vi "ajoutchambre.vi"() -> ()   [LabVIEW 2015]
uses:
  <vilib>/httpClient/LabVIEWHTTPClient.lvlib
panel:
  out "Tab Control 3":enum32{"Page 1", "Page 2"}(tab)
  out "Tab Control 2":enum32{"Page 1", "Page 2"}(tab)
  in  "desc":string
  in  "OK Button 4":bool
  in  "OK Button 2":bool
  out "Tab Control":enum32{"Page 1", "Page 2"}(tab)
  in  "nom":string
  in  "matricule":string
  # "Entrer Matricule"
  # "Entrer Nom"
  # "Entrer Description"
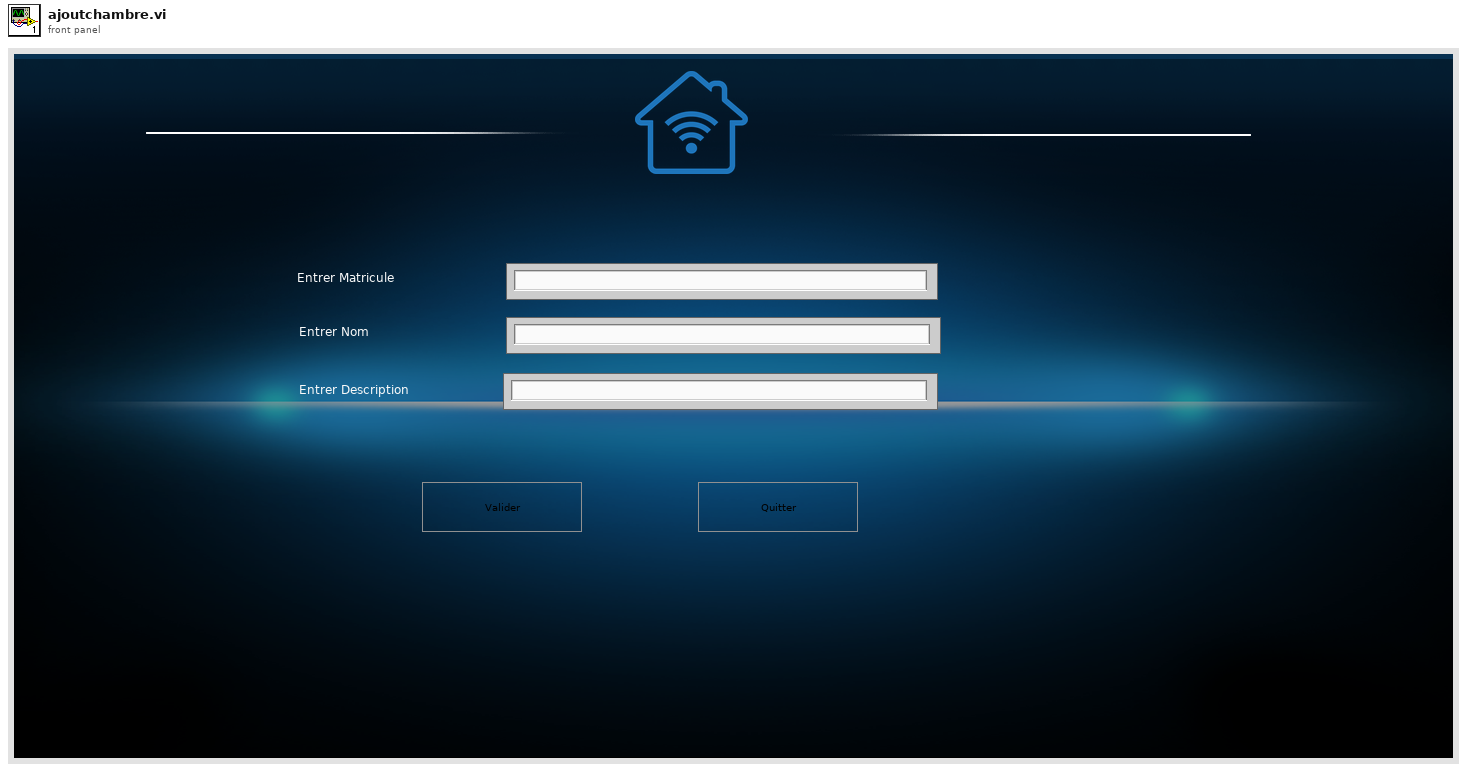
[diagram p1: front panel]
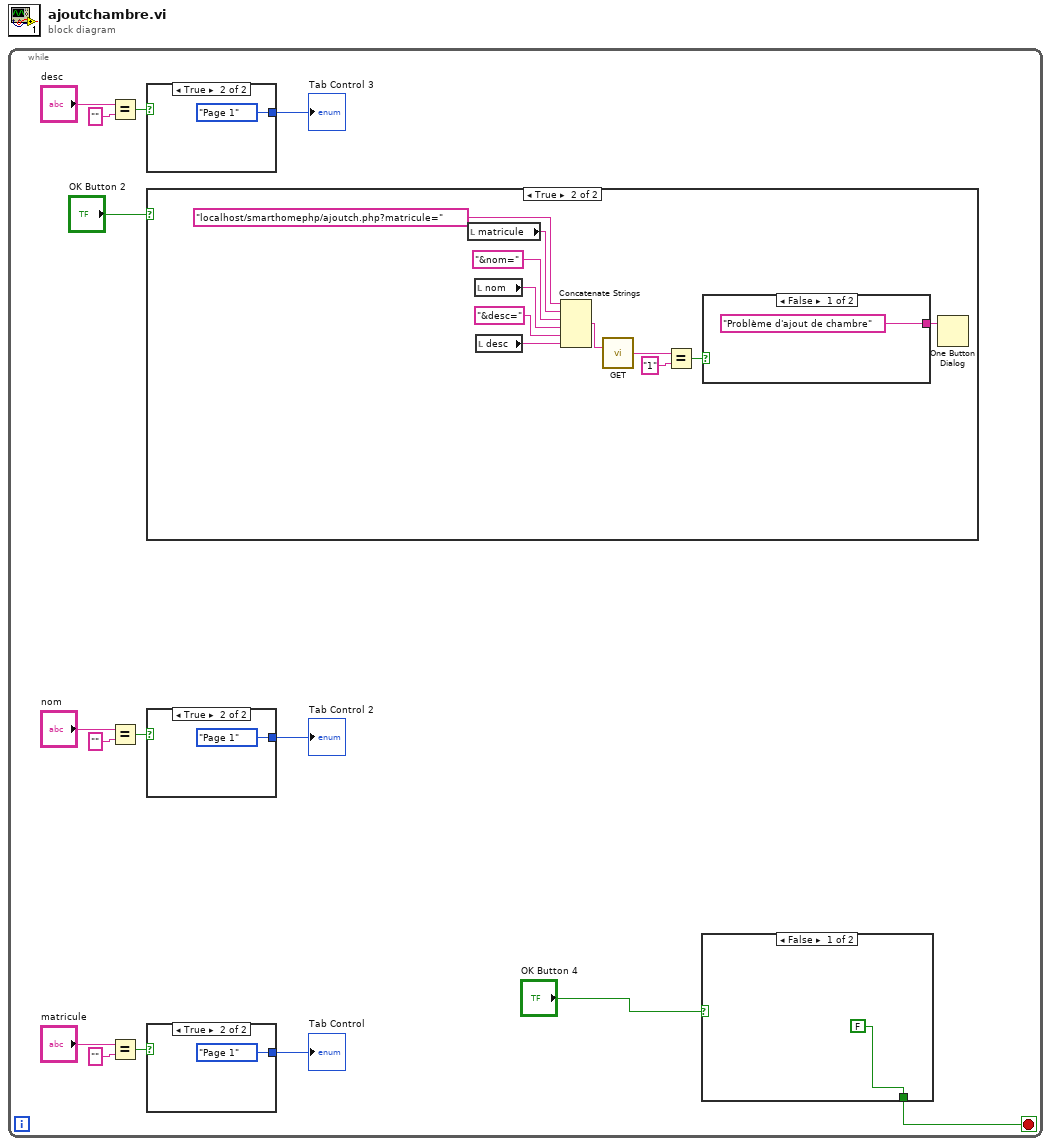
[diagram p0: block diagram]
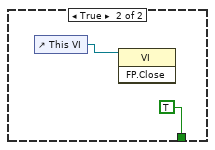
[diagram p2: hidden frame]
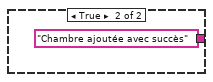
[diagram p4: hidden frame]
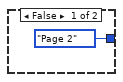
[diagram p5: hidden frame]
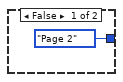
[diagram p6: hidden frame]
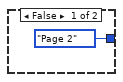
[diagram p7: hidden frame]
diagram:
  n1 = while {
    stop <- w1 stop-if-true
    n2 = Equal?(x="desc", y="") -> (x = y?=w5:bool)
    n3 = Equal?(x="nom", y="") -> (x = y?=w10:bool)
    n4 = Equal?(x="matricule", y="") -> (x = y?=w11:bool)
    n5 = case shown="True" w5 {
      tunnel: [enum32{"Page 1", "Page 2"}."Page 2" ("Tab Control") enum32{"Page 1", "Page 2"}."Page 1" ("Tab Control")] -> w4
      frame False {
      }
      frame True {
      }
    }
    "Tab Control 3" <- w4
    n6 = case shown="True" "OK Button 2" {
      frame False {
      }
      frame True {
        n7 = local read "matricule"() -> (w28:string)
        n8 = local read "nom"() -> (w26:string)
        n9 = local read "desc"() -> (w24:string)
        n10 = Concatenate Strings("localhost/smarthomephp/ajoutch.php?matricule=", w28, "&nom=", w26, "&desc=", w24) -> (w23:string)
        n11 = call <vilib>:"GET.vi"("url"=w23) -> ("body"=w22:string)  [unwired: 11 in, 3 out]
        n12 = Equal?(x=w22, y="1") -> (x = y?=w20:bool)
        n13 = case shown="False" w20 {
          tunnel: ["Problème d'ajout de chambre" "Chambre ajoutée avec succès"] -> w19
          frame False {
          }
          frame True {
          }
        }
        n14 = One Button Dialog(message=w19) -> ()  [unwired: 1 in, 1 out]
      }
    }
    n15 = case shown="True" w10 {
      tunnel: [enum32{"Page 1", "Page 2"}."Page 2" ("Tab Control") enum32{"Page 1", "Page 2"}."Page 1" ("Tab Control")] -> w8
      frame False {
      }
      frame True {
      }
    }
    "Tab Control 2" <- w8
    n16 = case shown="True" w11 {
      tunnel: [enum32{"Page 1", "Page 2"}."Page 2" ("Tab Control") enum32{"Page 1", "Page 2"}."Page 1" ("Tab Control")] -> w9
      frame False {
      }
      frame True {
      }
    }
    "Tab Control" <- w9
    n17 = case shown="False" "OK Button 4" {
      tunnel: [FALSE TRUE] -> w1
      frame False {
      }
      frame True {
        n18 = control-ref of="This VI"() -> (w18:refnum<vi>)
        n19 = invoke class="VI" method="FP.Close"(reference=w18) -> ()  [unwired: 2 in, 3 out]
      }
    }
  }
